vi "New.vi"(8 "error in (no error)":errorcluster, 11 "reference in":refnum<class "TestSuite_ImplementationFunctionality.lvclass">) -> (0 "error out":errorcluster, 3 "reference out":refnum<class "TestSuite_ImplementationFunctionality.lvclass">)   [LabVIEW 2013, in "TestSuite_ImplementationFunctionality.lvclass"]
uses:
  TestSuite_ImplementationFunctionality.lvclass
  <vilib>/addons/_JKI Toolkits/VI Tester/TestCase.llb/TestCase.lvclass
  TestSuite_ImplementationFunctionality.lvclass/TestSuite_ImplementationFunctionality.ctl
  <vilib>/addons/_JKI Toolkits/VI Tester/TestSuite.llb/TestSuite.lvclass
  Test Cases/ListImp_Common/ListImp_Common.lvclass
  source/LapDog.Collections.Lists.Implementations/BufferedArray/BufferedArray.lvclass
  Test Cases/ListImp_Empty/ListImp_Empty.lvclass
  Test Cases/ListImp_Populated/ListImp_Populated.lvclass
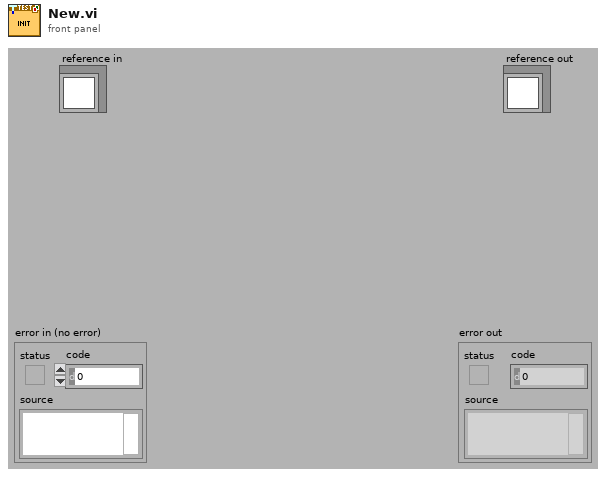
[diagram p1: front panel]
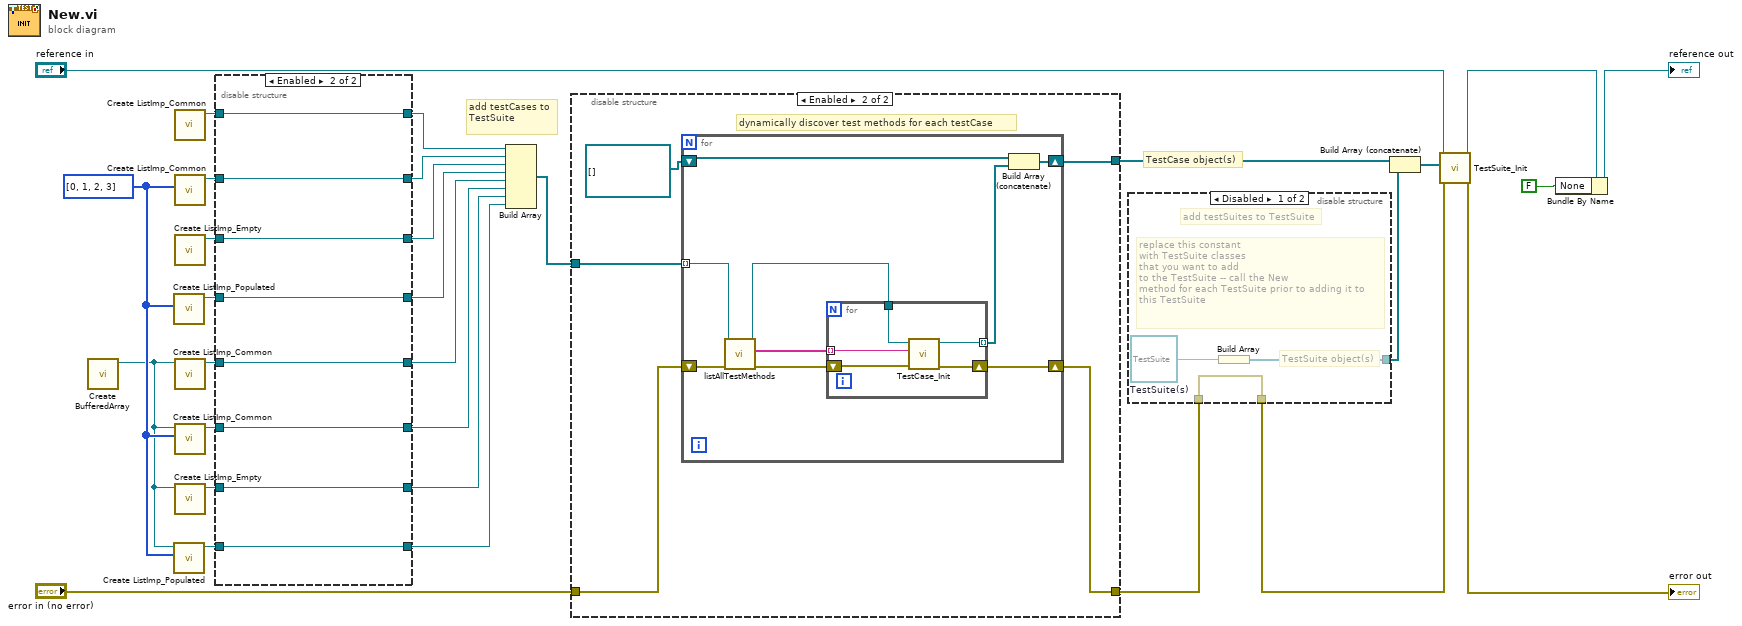
[diagram p0: block diagram]
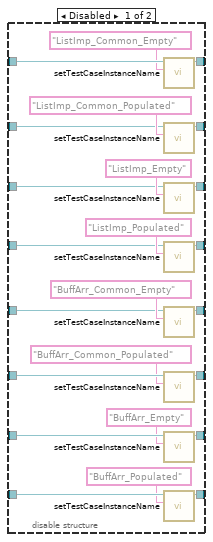
[diagram p2: hidden frame]
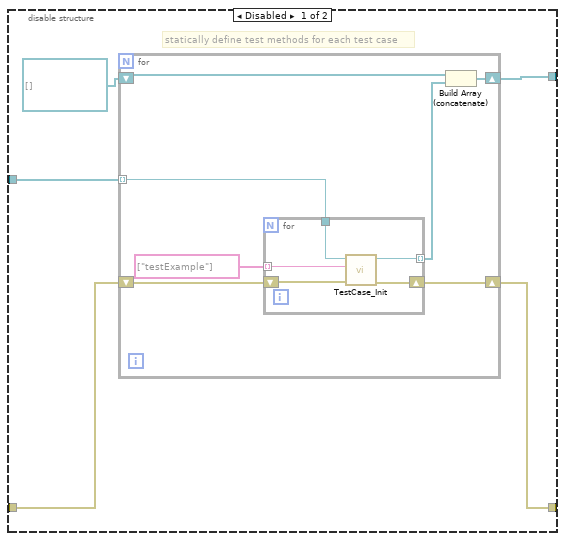
[diagram p4: hidden frame]
diagram:
  w6 = i32[] [0, 1, 2, 3] ("Initial List")
  # "TestCase object(s)"
  # "add testCases to TestSuite"
  n1 = call "Create BufferedArray.vi"() -> ("BufferedArray out"=w5:refnum<class "BufferedArray.lvclass">)  [unwired: 10 in, 1 out]
  n2 = call "Create ListImp_Populated.vi"("Initial List"=w6) -> ("ListImp_Populated out"=w12:refnum<class "ListImp_Populated.lvclass">)  [unwired: 9 in, 1 out]
  n3 = call "Create ListImp_Populated.vi"("Initial List"=w6, "ListImp"=w5) -> ("ListImp_Populated out"=w10:refnum<class "ListImp_Populated.lvclass">)  [unwired: 8 in, 1 out]
  n4 = call "Create ListImp_Common.vi"() -> ("ListImp_Reusable out"=w18:refnum<class "ListImp_Common.lvclass">)  [unwired: 10 in, 1 out]
  n5 = call "Create ListImp_Common.vi"("Initial List"=w6) -> ("ListImp_Reusable out"=w16:refnum<class "ListImp_Common.lvclass">)  [unwired: 9 in, 1 out]
  n6 = call "Create ListImp_Empty.vi"() -> ("ListImp_Empty out"=w14:refnum<class "ListImp_Empty.lvclass">)  [unwired: 10 in, 1 out]
  n7 = call "Create ListImp_Common.vi"("ListImp"=w5) -> ("ListImp_Reusable out"=w7:refnum<class "ListImp_Common.lvclass">)  [unwired: 9 in, 1 out]
  n8 = call "Create ListImp_Common.vi"("Initial List"=w6, "ListImp"=w5) -> ("ListImp_Reusable out"=w8:refnum<class "ListImp_Common.lvclass">)  [unwired: 8 in, 1 out]
  n9 = call "Create ListImp_Empty.vi"("ListImp"=w5) -> ("ListImp_Empty out"=w9:refnum<class "ListImp_Empty.lvclass">)  [unwired: 9 in, 1 out]
  n10 = disable-structure shown="Enabled" {
    disable-tunnel: w18 -> [w54 w62]
    disable-tunnel: [w53 w62] -> w17
    disable-tunnel: w16 -> [w50 w61]
    disable-tunnel: [w49 w61] -> w15
    disable-tunnel: w14 -> [w46 w60]
    disable-tunnel: [w45 w60] -> w13
    disable-tunnel: w12 -> [w44 w59]
    disable-tunnel: [w43 w59] -> w11
    disable-tunnel: w10 -> [w42 w55]
    disable-tunnel: w9 -> [w41 w56]
    disable-tunnel: w8 -> [w38 w57]
    disable-tunnel: w7 -> [w35 w58]
    disable-tunnel: [w34 w58] -> w4
    disable-tunnel: [w33 w57] -> w3
    disable-tunnel: [w32 w56] -> w2
    disable-tunnel: [w31 w55] -> w1
    frame Disabled {
      n11 = call <vilib>:"setTestCaseInstanceName.vi"("Test Case Instance Name (<Class Name>)"="ListImp_Common_Empty", "TestCase in"=w54) -> ("TestCase out"=w53:refnum<class "ListImp_Common.lvclass">)  [unwired: 9 in]
      n12 = call <vilib>:"setTestCaseInstanceName.vi"("Test Case Instance Name (<Class Name>)"="ListImp_Common_Populated", "TestCase in"=w50) -> ("TestCase out"=w49:refnum<class "ListImp_Common.lvclass">)  [unwired: 9 in]
      n13 = call <vilib>:"setTestCaseInstanceName.vi"("Test Case Instance Name (<Class Name>)"="ListImp_Empty", "TestCase in"=w46) -> ("TestCase out"=w45:refnum<class "ListImp_Empty.lvclass">)  [unwired: 9 in]
      n14 = call <vilib>:"setTestCaseInstanceName.vi"("Test Case Instance Name (<Class Name>)"="ListImp_Populated", "TestCase in"=w44) -> ("TestCase out"=w43:refnum<class "ListImp_Populated.lvclass">)  [unwired: 9 in]
      n15 = call <vilib>:"setTestCaseInstanceName.vi"("Test Case Instance Name (<Class Name>)"="BuffArr_Common_Empty", "TestCase in"=w35) -> ("TestCase out"=w34:refnum<class "ListImp_Common.lvclass">)  [unwired: 9 in]
      n16 = call <vilib>:"setTestCaseInstanceName.vi"("Test Case Instance Name (<Class Name>)"="BuffArr_Common_Populated", "TestCase in"=w38) -> ("TestCase out"=w33:refnum<class "ListImp_Common.lvclass">)  [unwired: 9 in]
      n17 = call <vilib>:"setTestCaseInstanceName.vi"("Test Case Instance Name (<Class Name>)"="BuffArr_Empty", "TestCase in"=w41) -> ("TestCase out"=w32:refnum<class "ListImp_Empty.lvclass">)  [unwired: 9 in]
      n18 = call <vilib>:"setTestCaseInstanceName.vi"("Test Case Instance Name (<Class Name>)"="BuffArr_Populated", "TestCase in"=w42) -> ("TestCase out"=w31:refnum<class "ListImp_Populated.lvclass">)  [unwired: 9 in]
    }
    frame Enabled {
    }
  }
  n19 = Build Array(w17, w15, w13, w11, w4, w3, w2, w1) -> (w24:refnum<class "TestCase.lvclass">[])
  n20 = disable-structure shown="Enabled" {
    disable-tunnel: w24 -> [w67 w84]
    disable-tunnel: "error in (no error)" -> [w65 w82]
    disable-tunnel: [w64 w81] -> w23
    disable-tunnel: [w63 w80] -> w19
    frame Disabled {
      # "statically define test methods for each test case"
      n21 = for {
        shift-right: [w72] -> w63
        shift-left: w65 -> [w73]
        tunnel: w67 -> [w71] mode=indexing
        shift-right: [w68] -> w64
        shift-left: refnum<class "TestCase.lvclass">[] [] -> [w69]
        n22 = for {
          tunnel: w71 -> [w75]
          tunnel: string[] ["testExample"] ("tests") -> [w79] mode=indexing
          shift-right: [w77] -> w72
          shift-left: w73 -> [w78]
          tunnel: [w76] -> w70 mode=indexing
          n23 = call <vilib>:"TestCase_Init.vi"("error in (no error)"=w78, "methodName (\"runTest\")"=w79, "TestCase in"=w75) -> ("error out"=w77:errorcluster, "TestCase out"=w76:refnum<class "TestCase.lvclass">)  [unwired: 7 in]
        }
        n24 = Build Array (concatenate)(w69, w70) -> (w68:refnum<class "TestCase.lvclass">[])
      }
    }
    frame Enabled {
      # "dynamically discover test methods for each testCase"
      n25 = for {
        shift-right: [w93] -> w80
        shift-left: w82 -> [w89]
        tunnel: w84 -> [w86] mode=indexing
        shift-right: [w90] -> w81
        shift-left: refnum<class "TestCase.lvclass">[] [] -> [w91]
        n26 = call-dynamic "listAllTestMethods.vi"("error in (no error)"=w89, "TestCase in"=w86) -> ("error out"=w88:errorcluster, "test methods"=w87:string[], "TestCase out"=w85:refnum<class "TestCase.lvclass">)  [unwired: 7 in]
        n27 = for {
          tunnel: w85 -> [w94]
          tunnel: w87 -> [w98] mode=indexing
          shift-right: [w96] -> w93
          shift-left: w88 -> [w97]
          tunnel: [w95] -> w92 mode=indexing
          n28 = call <vilib>:"TestCase_Init.vi"("error in (no error)"=w97, "methodName (\"runTest\")"=w98, "TestCase in"=w94) -> ("error out"=w96:errorcluster, "TestCase out"=w95:refnum<class "TestCase.lvclass">)  [unwired: 7 in]
        }
        n29 = Build Array (concatenate)(w91, w92) -> (w90:refnum<class "TestCase.lvclass">[])
      }
    }
  }
  n30 = disable-structure shown="Disabled" {
    disable-tunnel: [w99 _] -> w21
    disable-tunnel: [w101 w102] -> w20
    disable-tunnel: w19 -> [w101 w102]
    frame Disabled {
      w100 = refnum<class "TestSuite.lvclass"> refnum  # TestSuite(s)
      # "replace this constant\nwith TestSuite classes\nthat you want to add\nto the TestSuite -- call the New\nmethod for each TestSuite prior to adding it to\nthis TestSuite"
      # "add testSuites to TestSuite"
      # "TestSuite object(s)"
      n31 = Build Array(w100) -> (w99:refnum<class "TestSuite.lvclass">[])
    }
    frame Enabled {
    }
  }
  n32 = Build Array (concatenate)(w23, w21) -> (w22:refnum<class>[])
  n33 = call <vilib>:"TestSuite_Init.vi"("error in (no error)"=w20, "tests (none)"=w22, "TestSuite in"="reference in") -> ("error out"=→"error out":errorcluster, "TestSuite out"=w25:refnum<class "TestSuite_ImplementationFunctionality.lvclass">)  [unwired: 7 in]
  n34 = Bundle By Name(cluster=w25, "None"=FALSE) -> (→"reference out":refnum<class "TestSuite_ImplementationFunctionality.lvclass">)
